vi "Semaforo.vi"() -> ()   [LabVIEW 2018]
panel:
  out "?":cluster{bool, bool, bool}
  in  "?":bool
  out "?":cluster{bool, bool, bool}
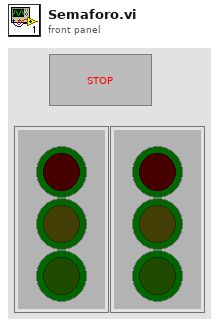
[diagram p1: front panel]
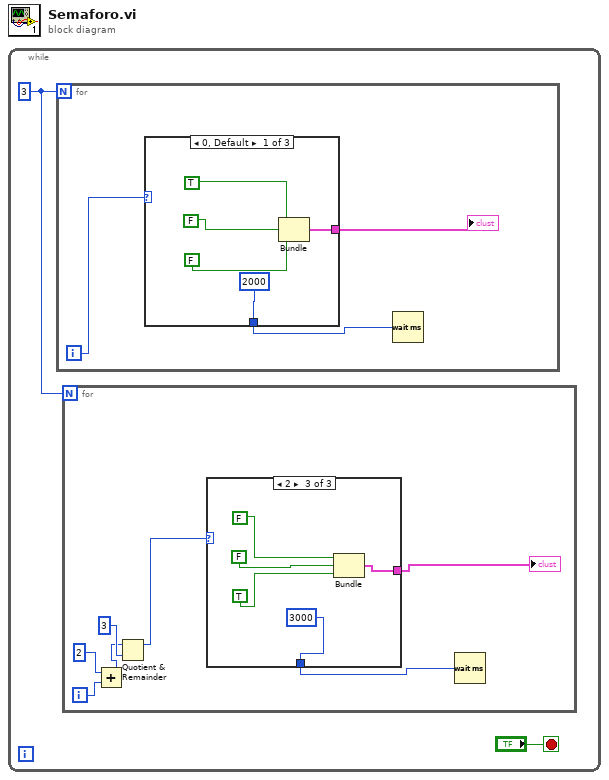
[diagram p0: block diagram]
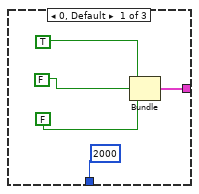
[diagram p2: hidden frame]
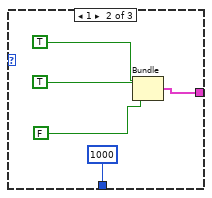
[diagram p3: hidden frame]
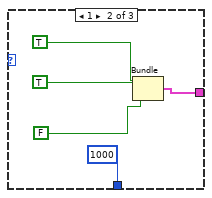
[diagram p4: hidden frame]
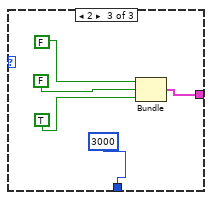
[diagram p5: hidden frame]
diagram:
  n1 = while {
    stop <- "?" stop-if-true
    w1 = 3
    n2 = for {
      N: w1 -> [_]
      i -> [w25]
      n3 = case shown="0, Default" w25 {
        tunnel: [u32 2000 ("milliseconds to wait") u32 1000 ("milliseconds to wait") u32 3000 ("milliseconds to wait")] -> w27
        tunnel: [w28 w33 w38] -> w26
        frame 0, Default {
          n4 = Bundle(TRUE, FALSE, FALSE) -> (w28:cluster{bool, bool, bool})  [unwired: 1 in]
        }
        frame 1 {
          n5 = Bundle(TRUE, TRUE, FALSE) -> (w33:cluster{bool, bool, bool})  [unwired: 1 in]
        }
        frame 2 {
          n6 = Bundle(FALSE, FALSE, TRUE) -> (w38:cluster{bool, bool, bool})  [unwired: 1 in]
        }
      }
      "?" <- w26
      n7 = Wait (ms)(milliseconds to wait=w27) -> ()  [unwired: 1 out]
    }
    n8 = for {
      N: w1 -> [_]
      i -> [w5]
      n9 = Add(x=2 ("y"), y=w5) -> (x+y=w4:i32)
      n10 = Quotient & Remainder(x=w4, y=3) -> (x-y*floor(x/y)=w3:i32)  [unwired: 1 out]
      n11 = case shown="2" w3 {
        tunnel: [u32 2000 ("milliseconds to wait") u32 1000 ("milliseconds to wait") u32 3000 ("milliseconds to wait")] -> w8
        tunnel: [w10 w15 w20] -> w9
        frame 0, Default {
          n12 = Bundle(TRUE, FALSE, FALSE) -> (w10:cluster{bool, bool, bool})  [unwired: 1 in]
        }
        frame 1 {
          n13 = Bundle(TRUE, TRUE, FALSE) -> (w15:cluster{bool, bool, bool})  [unwired: 1 in]
        }
        frame 2 {
          n14 = Bundle(FALSE, FALSE, TRUE) -> (w20:cluster{bool, bool, bool})  [unwired: 1 in]
        }
      }
      "?" <- w9
      n15 = Wait (ms)(milliseconds to wait=w8) -> ()  [unwired: 1 out]
    }
  }
